vi "Process EMS Message.vi"(8 "error in (no error)":errorcluster, 10 "EMS Message":T1, 11 "Master Controller in":refnum<class "Master Controller.lvclass">) -> (0 "error out":errorcluster, 3 "Master Controller out":refnum<class "Master Controller.lvclass">)   [LabVIEW 2015, in "Master Controller Core.lvlib" / "Master Controller.lvclass"]
uses:
  Master Controller.lvclass
  Communications/SCADA Communcations Actor/SCADA Communications/Controls/EMS Message Cluster.ctl
  Master Controller.lvclass/Master Controller.ctl
  Communications/SCADA Communcations Actor/SCADA Communications Messages/Transmit EMS Message Msg/Transmit EMS Message Msg.lvclass/Transmit EMS Message Msg.ctl
  <vilib>/ActorFramework/Message Enqueuer/Message Enqueuer.lvclass/Message Enqueuer.ctl
  SCADA Core/SCADA Action Messages/Black Start Msg/Black Start Msg.lvclass/Black Start Msg.ctl
  <vilib>/ActorFramework/Actor/Actor.lvclass/Actor.ctl
  Master Controller Messages/Save CID File Msg/Save CID File Msg.lvclass/Save CID File Msg.ctl
  SCADA Core/SCADA Action Messages/Device Load Msg/Device Load Msg.lvclass/Device Load Msg.ctl
  SCADA Core/SCADA Action Messages/Device Unload Msg/Device Unload Msg.lvclass/Device Unload Msg.ctl
  IED Actor/IED/Controls/Device Activate Mode Select.ctl
  SCADA Core/SCADA Action Messages/Device Activate Msg/Device Activate Msg.lvclass/Device Activate Msg.ctl
  SCADA Core/SCADA Action Messages/Device Deactivate Msg/Device Deactivate Msg.lvclass/Device Deactivate Msg.ctl
  SCADA Core/SCADA Action Messages/Get Device Parameter Msg/Get Device Parameter Msg.lvclass/Get Device Parameter Msg.ctl
  SCADA Core/SCADA Action Messages/Set Device Parameter Msg/Set Device Parameter Msg.lvclass/Set Device Parameter Msg.ctl
  SCADA Core/SCADA Action Messages/Island Control Msg/Island Control Msg.lvclass/Island Control Msg.ctl
  SCADA Core/SCADA Action Messages/Get Measurement Msg/Get Measurement Msg.lvclass/Get Measurement Msg.ctl
  SCADA Core/SCADA Action Messages/Get Measurement (Multiple) Msg/Get Measurement (Multiple) Msg.lvclass/Get Measurement (Multiple) Msg.ctl
  SCADA Core/SCADA Action Messages/PCC Relay Msg/PCC Relay Msg.lvclass/PCC Relay Msg.ctl
  SCADA Core/SCADA Action Messages/Write Setpoint (Multiple) Msg/Write Setpoint (Multiple) Msg.lvclass/Write Setpoint (Multiple) Msg.ctl
  SCADA Core/SCADA Action Messages/Write Setpoint Msg/Write Setpoint Msg.lvclass/Write Setpoint Msg.ctl
  <vilib>/ActorFramework/Message Enqueuer/Enqueue.vi
  <vilib>/ActorFramework/Message Enqueuer/Init from Existing Queue.vi
  <vilib>/ActorFramework/Message Priority Queue/Priority Enqueue.vi
  Communications/SCADA Communcations Actor/SCADA Communications Messages/Transmit EMS Message Msg/Transmit EMS Message Msg.lvclass
  SCADA Core/SCADA Action Messages/Activate Msg/Activate Msg.lvclass
  SCADA Core/SCADA Action Messages/Black Start Msg/Black Start Msg.lvclass
  <vilib>/ActorFramework/Message Enqueuer/Message Enqueuer.lvclass
  Master Controller Messages/Save CID File Msg/Save CID File Msg.lvclass
  SCADA Core/SCADA Action Messages/Device Load Msg/Device Load Msg.lvclass
  SCADA Core/SCADA Action Messages/Device Unload Msg/Device Unload Msg.lvclass
  SCADA Core/SCADA Action Messages/Device Activate Msg/Device Activate Msg.lvclass
  SCADA Core/SCADA Action Messages/Device Deactivate Msg/Device Deactivate Msg.lvclass
  SCADA Core/SCADA Action Messages/Get Device Parameter Msg/Get Device Parameter Msg.lvclass
  SCADA Core/SCADA Action Messages/Set Device Parameter Msg/Set Device Parameter Msg.lvclass
  SCADA Core/SCADA Action Messages/Island Control Msg/Island Control Msg.lvclass
  SCADA Core/SCADA Action Messages/Get Measurement Msg/Get Measurement Msg.lvclass
  SCADA Core/SCADA Action Messages/Get Measurement (Multiple) Msg/Get Measurement (Multiple) Msg.lvclass
  SCADA Core/SCADA Action Messages/PCC Relay Msg/PCC Relay Msg.lvclass
  SCADA Core/SCADA Action Messages/Write Setpoint (Multiple) Msg/Write Setpoint (Multiple) Msg.lvclass
  SCADA Core/SCADA Action Messages/Write Setpoint Msg/Write Setpoint Msg.lvclass
  SCADA Core/SCADA Action Messages/Shutdown Msg/Shutdown Msg.lvclass
  SCADA Core/SCADA Action Messages/Synchronize Msg/Synchronize Msg.lvclass
  SCADA Core/SCADA Messages/Island Msg/Island Msg.lvclass
  Communications/SCADA Communcations Actor/SCADA Communications/SCADA Communications.lvclass
  <vilib>/ActorFramework/Actor/Actor.lvclass
  Utilities/Message Strings.llb/Message String Utilities.lvlib
  IED Actor/IED/IED.lvclass
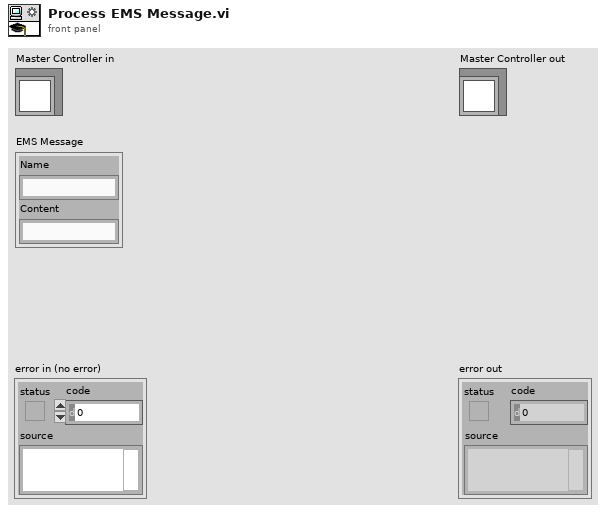
[diagram p1: front panel]
types:
  T1 = typedef "SCADA Communcations Actor.lvlib/SCADA Communications.lvclass/EMS Message Cluster.ctl" = cluster{"Name":string, "Content":string}
  T2 = typedef "IED Actor.lvlib/IED.lvclass/Device Activate Mode Select.ctl" = enum16{"Activate", "Blackstart", "Individual"}
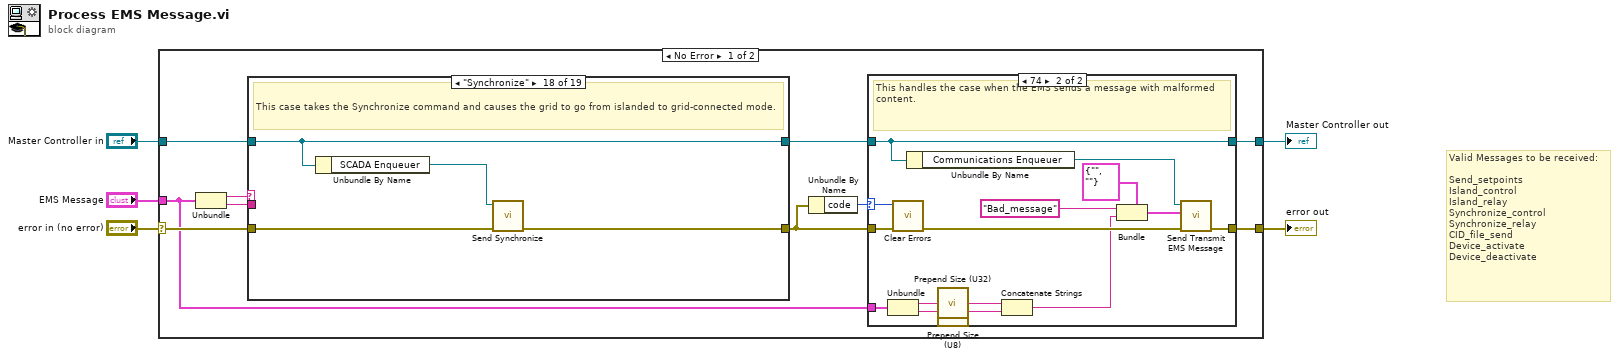
[diagram p0: block diagram]
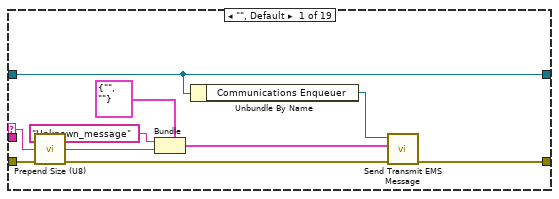
[diagram p3: hidden frame]
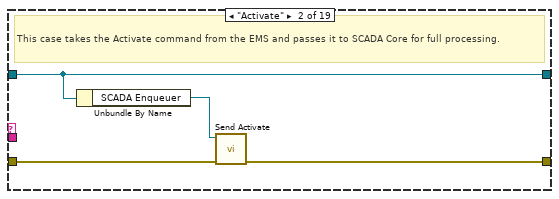
[diagram p4: hidden frame]
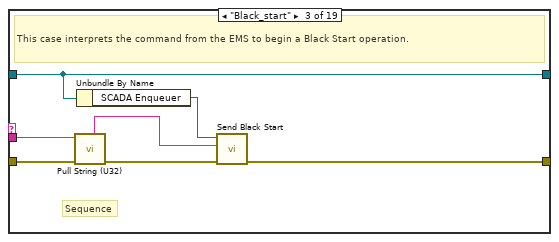
[diagram p5: hidden frame]
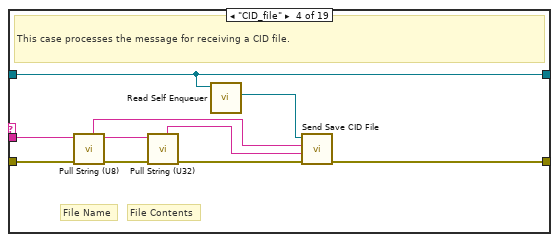
[diagram p6: hidden frame]
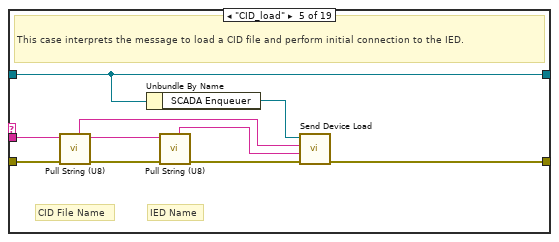
[diagram p7: hidden frame]
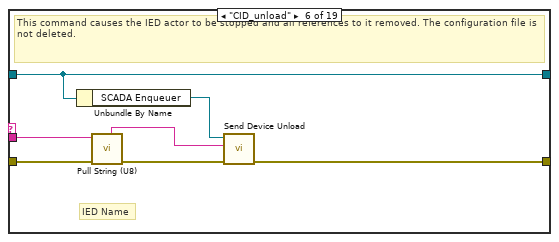
[diagram p8: hidden frame]
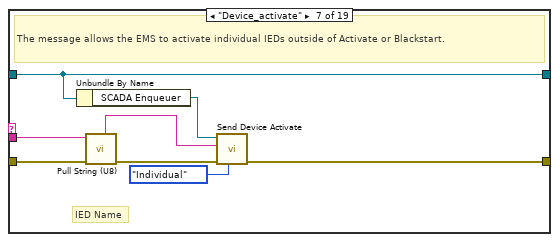
[diagram p9: hidden frame]
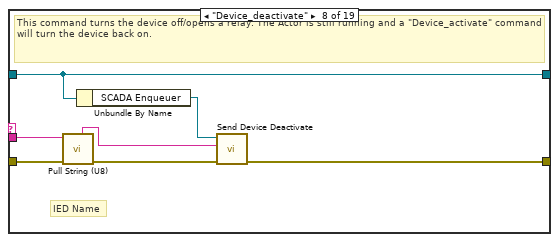
[diagram p10: hidden frame]
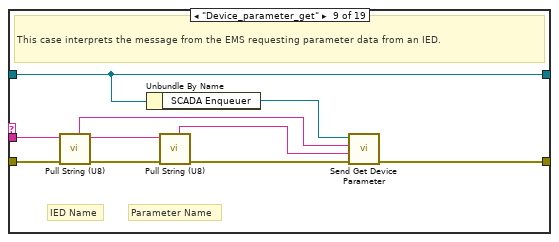
[diagram p11: hidden frame]
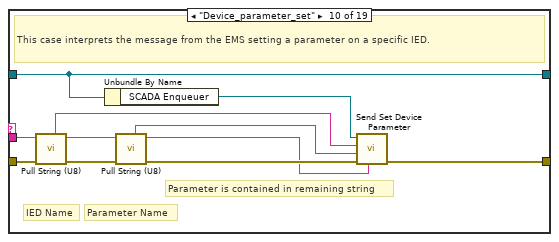
[diagram p12: hidden frame]
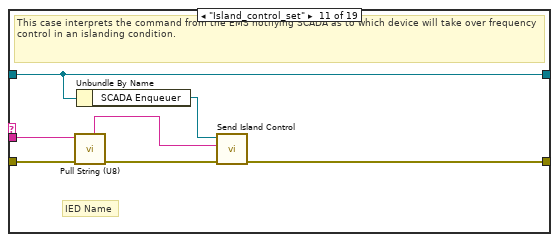
[diagram p13: hidden frame]
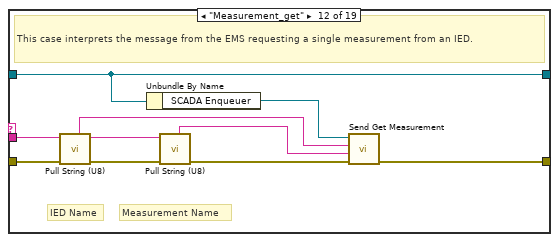
[diagram p14: hidden frame]
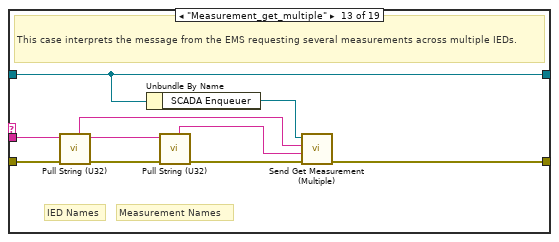
[diagram p15: hidden frame]
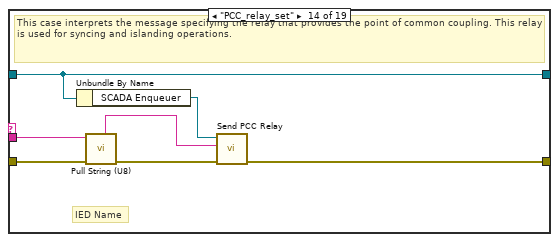
[diagram p16: hidden frame]
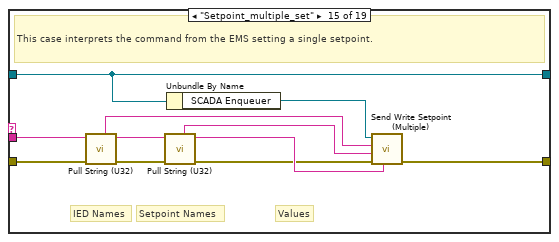
[diagram p17: hidden frame]
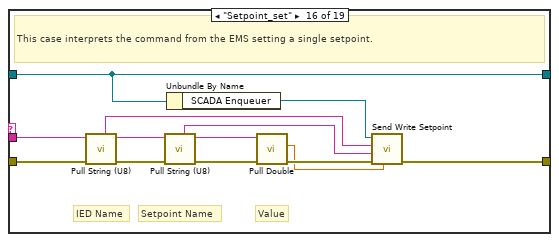
[diagram p18: hidden frame]
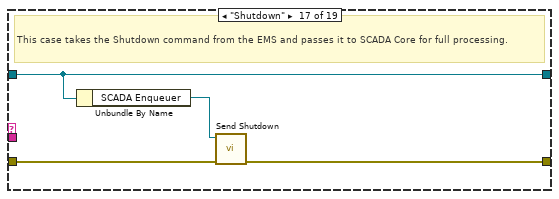
[diagram p19: hidden frame]
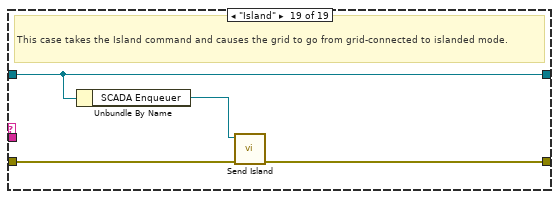
[diagram p20: hidden frame]
diagram:
  # "Valid Messages to be received:\n\nSend_setpoints\nIsland_control\nIsland_relay\nSynchronize_control\nSynchronize_relay\nCID_file_send\nDevice_activate\nDevice_deactivate"
  n1 = case shown="No Error" "error in (no error)" {
    selector: "error in (no error)" -> [w12 w187]
    tunnel: [w10 w187] -> w4
    tunnel: [w6 w186] -> w2
    tunnel: "Master Controller in" -> [w15 w186]
    tunnel: "EMS Message" -> [w8 _]
    frame No Error {
      n2 = Unbundle(w8) -> ("Name"=w14:string, "Content"=w13:string)
      n3 = case shown="\"Synchronize\"" w14 {
        selector: w14 -> [w35 _ _ _ _ _ _ _ _ _ _ _ _ _ _ _ _ _ _]
        tunnel: w15 -> [w41 w45 w52 w62 w72 w79 w87 w94 w104 w115 w122 w132 w142 w149 w160 w173 w177 w181 w185]
        tunnel: w13 -> [_ _ w49 w59 w68 w76 w84 w90 w102 w113 w119 w130 w140 w146 w157 w170 _ _ _]
        tunnel: [w41 w45 w52 w62 w72 w79 w87 w94 w104 w115 w122 w132 w142 w149 w160 w173 w177 w181 w185] -> w7
        tunnel: w12 -> [w36 w42 w48 w58 w69 w75 w83 w91 w103 w114 w118 w131 w141 w145 w156 w169 w174 w179 w183]
        tunnel: [w37 w43 w50 w60 w70 w78 w85 w92 w97 w108 w120 w125 w136 w147 w158 w171 w175 w178 w182] -> w9
        frame "", Default {
          n4 = call "Prepend Size (U8).vi"("String in"=w35) -> ("String out"=w33:string)
          n5 = Bundle(cluster=T1 {"Name"="", "Content"=""} ("Message"), "Name"="Unknown_message", "Content"=w33) -> (w38:T1)
          n6 = Unbundle By Name(w41) -> ("Communications Enqueuer"=w40:refnum<class "Message Enqueuer.lvclass">)
          n7 = call "Send Transmit EMS Message.vi"("error in (no error)"=w36, "Message"=w38, "Message Enqueuer"=w40) -> ("error out"=w37:errorcluster)  [unwired: 7 in, 1 out]
        }
        frame "Activate" {
          # "This case takes the Activate command from the EMS and passes it to SCADA Core for full processing."
          n8 = Unbundle By Name(w45) -> ("SCADA Enqueuer"=w44:refnum<class "Message Enqueuer.lvclass">)
          n9 = call "Send Activate.vi"("error in (no error)"=w42, "Message Enqueuer"=w44) -> ("error out"=w43:errorcluster)  [unwired: 8 in, 1 out]
        }
        frame "Black_start" {
          # "Sequence"
          # "This case interprets the command from the EMS to begin a Black Start operation."
          n10 = call "Pull String (U32).vi"("error in (no error)"=w48, "String in"=w49) -> ("error out"=w47:errorcluster, "String out"=w46:string)  [unwired: 7 in, 1 out]
          n11 = Unbundle By Name(w52) -> ("SCADA Enqueuer"=w51:refnum<class "Message Enqueuer.lvclass">)
          n12 = call "Send Black Start.vi"("error in (no error)"=w47, "Sequence"=w46, "Message Enqueuer"=w51) -> ("error out"=w50:errorcluster)  [unwired: 7 in, 1 out]
        }
        frame "CID_file" {
          # "File Contents"
          # "File Name"
          # "This case processes the message for receiving a CID file."
          n13 = call "Pull String (U8).vi"("error in (no error)"=w58, "String in"=w59) -> ("error out"=w56:errorcluster, "Remaining String"=w57:string, "String out"=w53:string)  [unwired: 7 in]
          n14 = call "Pull String (U32).vi"("error in (no error)"=w56, "String in"=w57) -> ("error out"=w55:errorcluster, "String out"=w54:string)  [unwired: 7 in, 1 out]
          n15 = call <vilib>:"Read Self Enqueuer.vi"("Actor"=w62) -> ("Self Enqueuer"=w61:refnum<class "Message Enqueuer.lvclass">)  [unwired: 10 in]
          n16 = call "Send Save CID File.vi"("error in (no error)"=w55, "Content"=w54, "File Name"=w53, "Message Enqueuer"=w61) -> ("error out"=w60:errorcluster)  [unwired: 6 in, 1 out]
        }
        frame "CID_load" {
          # "IED Name"
          # "CID File Name"
          # "This case interprets the message to load a CID file and perform initial connection to the IED."
          n17 = call "Pull String (U8).vi"("error in (no error)"=w69, "String in"=w68) -> ("error out"=w67:errorcluster, "Remaining String"=w63:string, "String out"=w65:string)  [unwired: 7 in]
          n18 = Unbundle By Name(w72) -> ("SCADA Enqueuer"=w71:refnum<class "Message Enqueuer.lvclass">)
          n19 = call "Pull String (U8).vi"("error in (no error)"=w67, "String in"=w63) -> ("error out"=w66:errorcluster, "String out"=w64:string)  [unwired: 7 in, 1 out]
          n20 = call "Send Device Load.vi"("error in (no error)"=w66, "IED Name"=w64, "CID File Name"=w65, "Message Enqueuer"=w71) -> ("error out"=w70:errorcluster)  [unwired: 6 in, 1 out]
        }
        frame "CID_unload" {
          # "IED Name"
          # "This command causes the IED actor to be stopped and all references to it removed. The configuration file is not deleted."
          n21 = Unbundle By Name(w79) -> ("SCADA Enqueuer"=w77:refnum<class "Message Enqueuer.lvclass">)
          n22 = call "Pull String (U8).vi"("error in (no error)"=w75, "String in"=w76) -> ("error out"=w74:errorcluster, "String out"=w73:string)  [unwired: 7 in, 1 out]
          n23 = call "Send Device Unload.vi"("error in (no error)"=w74, "IED Name"=w73, "Message Enqueuer"=w77) -> ("error out"=w78:errorcluster)  [unwired: 7 in, 1 out]
        }
        frame "Device_activate" {
          # "IED Name"
          # "The message allows the EMS to activate individual IEDs outside of Activate or Blackstart."
          n24 = Unbundle By Name(w87) -> ("SCADA Enqueuer"=w86:refnum<class "Message Enqueuer.lvclass">)
          n25 = call "Pull String (U8).vi"("error in (no error)"=w83, "String in"=w84) -> ("error out"=w82:errorcluster, "String out"=w81:string)  [unwired: 7 in, 1 out]
          n26 = call "Send Device Activate.vi"("Activate Mode"=Device_Activate_Mode_Select."Individual", "error in (no error)"=w82, "IED Name"=w81, "Message Enqueuer"=w86) -> ("error out"=w85:errorcluster)  [unwired: 6 in, 1 out]
        }
        frame "Device_deactivate" {
          # "IED Name"
          # "This command turns the device off/opens a relay. The Actor is still running and a \"Device_activate\" command will turn the device back on."
          n27 = call "Pull String (U8).vi"("error in (no error)"=w91, "String in"=w90) -> ("error out"=w89:errorcluster, "String out"=w88:string)  [unwired: 7 in, 1 out]
          n28 = Unbundle By Name(w94) -> ("SCADA Enqueuer"=w93:refnum<class "Message Enqueuer.lvclass">)
          n29 = call "Send Device Deactivate.vi"("error in (no error)"=w89, "IED Name"=w88, "Message Enqueuer"=w93) -> ("error out"=w92:errorcluster)  [unwired: 7 in, 1 out]
        }
        frame "Device_parameter_get" {
          # "Parameter Name"
          # "IED Name"
          # "This case interprets the message from the EMS requesting parameter data from an IED."
          n30 = call "Pull String (U8).vi"("error in (no error)"=w103, "String in"=w102) -> ("error out"=w101:errorcluster, "Remaining String"=w100:string, "String out"=w95:string)  [unwired: 7 in]
          n31 = Unbundle By Name(w104) -> ("SCADA Enqueuer"=w99:refnum<class "Message Enqueuer.lvclass">)
          n32 = call "Pull String (U8).vi"("error in (no error)"=w101, "String in"=w100) -> ("error out"=w98:errorcluster, "String out"=w96:string)  [unwired: 7 in, 1 out]
          n33 = call "Send Get Device Parameter.vi"("error in (no error)"=w98, "Parameter Name"=w96, "IED Name"=w95, "Message Enqueuer"=w99) -> ("error out"=w97:errorcluster)  [unwired: 6 in, 1 out]
        }
        frame "Device_parameter_set" {
          # "Parameter is contained in remaining string"
          # "Parameter Name"
          # "IED Name"
          # "This case interprets the message from the EMS setting a parameter on a specific IED."
          n34 = call "Pull String (U8).vi"("error in (no error)"=w114, "String in"=w113) -> ("error out"=w112:errorcluster, "Remaining String"=w111:string, "String out"=w106:string)  [unwired: 7 in]
          n35 = Unbundle By Name(w115) -> ("SCADA Enqueuer"=w110:refnum<class "Message Enqueuer.lvclass">)
          n36 = call "Pull String (U8).vi"("error in (no error)"=w112, "String in"=w111) -> ("error out"=w109:errorcluster, "Remaining String"=w105:string, "String out"=w107:string)  [unwired: 7 in]
          n37 = call "Send Set Device Parameter.vi"("Parameter"=w105, "error in (no error)"=w109, "Parameter Name"=w107, "IED Name"=w106, "Message Enqueuer"=w110) -> ("error out"=w108:errorcluster)  [unwired: 5 in, 1 out]
        }
        frame "Island_control_set" {
          # "IED Name"
          # "This case interprets the command from the EMS notifying SCADA as to which device will take over frequency control in an islanding condition."
          n38 = call "Pull String (U8).vi"("error in (no error)"=w118, "String in"=w119) -> ("error out"=w117:errorcluster, "String out"=w116:string)  [unwired: 7 in, 1 out]
          n39 = Unbundle By Name(w122) -> ("SCADA Enqueuer"=w121:refnum<class "Message Enqueuer.lvclass">)
          n40 = call "Send Island Control.vi"("error in (no error)"=w117, "IED Name"=w116, "Message Enqueuer"=w121) -> ("error out"=w120:errorcluster)  [unwired: 7 in, 1 out]
        }
        frame "Measurement_get" {
          # "Measurement Name"
          # "IED Name"
          # "This case interprets the message from the EMS requesting a single measurement from an IED."
          n41 = call "Pull String (U8).vi"("error in (no error)"=w131, "String in"=w130) -> ("error out"=w129:errorcluster, "Remaining String"=w128:string, "String out"=w123:string)  [unwired: 7 in]
          n42 = Unbundle By Name(w132) -> ("SCADA Enqueuer"=w127:refnum<class "Message Enqueuer.lvclass">)
          n43 = call "Pull String (U8).vi"("error in (no error)"=w129, "String in"=w128) -> ("error out"=w126:errorcluster, "String out"=w124:string)  [unwired: 7 in, 1 out]
          n44 = call "Send Get Measurement.vi"("error in (no error)"=w126, "Measurement Name"=w124, "IED Name"=w123, "Message Enqueuer"=w127) -> ("error out"=w125:errorcluster)  [unwired: 6 in, 1 out]
        }
        frame "Measurement_get_multiple" {
          # "Measurement Names"
          # "IED Names"
          # "This case interprets the message from the EMS requesting several measurements across multiple IEDs."
          n45 = call "Pull String (U32).vi"("error in (no error)"=w141, "String in"=w140) -> ("error out"=w139:errorcluster, "Remaining String"=w138:string, "String out"=w134:string)  [unwired: 7 in]
          n46 = Unbundle By Name(w142) -> ("SCADA Enqueuer"=w135:refnum<class "Message Enqueuer.lvclass">)
          n47 = call "Pull String (U32).vi"("error in (no error)"=w139, "String in"=w138) -> ("error out"=w137:errorcluster, "String out"=w133:string)  [unwired: 7 in, 1 out]
          n48 = call "Send Get Measurement (Multiple).vi"("error in (no error)"=w137, "Measurement Names"=w133, "IED Names"=w134, "Message Enqueuer"=w135) -> ("error out"=w136:errorcluster)  [unwired: 6 in, 1 out]
        }
        frame "PCC_relay_set" {
          # "IED Name"
          # "This case interprets the message specifying the relay that provides the point of common coupling. This relay is used for syncing and islanding operations."
          n49 = Unbundle By Name(w149) -> ("SCADA Enqueuer"=w148:refnum<class "Message Enqueuer.lvclass">)
          n50 = call "Pull String (U8).vi"("error in (no error)"=w145, "String in"=w146) -> ("error out"=w144:errorcluster, "String out"=w143:string)  [unwired: 7 in, 1 out]
          n51 = call "Send PCC Relay.vi"("error in (no error)"=w144, "Relay Name"=w143, "Message Enqueuer"=w148) -> ("error out"=w147:errorcluster)  [unwired: 7 in, 1 out]
        }
        frame "Setpoint_multiple_set" {
          # "Values"
          # "Setpoint Names"
          # "IED Names"
          # "This case interprets the command from the EMS setting a single setpoint."
          n52 = call "Pull String (U32).vi"("error in (no error)"=w156, "String in"=w157) -> ("error out"=w155:errorcluster, "Remaining String"=w154:string, "String out"=w152:string)  [unwired: 7 in]
          n53 = call "Pull String (U32).vi"("error in (no error)"=w155, "String in"=w154) -> ("error out"=w150:errorcluster, "Remaining String"=w151:string, "String out"=w153:string)  [unwired: 7 in]
          n54 = Unbundle By Name(w160) -> ("SCADA Enqueuer"=w159:refnum<class "Message Enqueuer.lvclass">)
          n55 = call "Send Write Setpoint (Multiple).vi"("Values"=w151, "error in (no error)"=w150, "Variables"=w153, "IED Names"=w152, "Message Enqueuer"=w159) -> ("error out"=w158:errorcluster)  [unwired: 5 in, 1 out]
        }
        frame "Setpoint_set" {
          # "Value"
          # "Setpoint Name"
          # "IED Name"
          # "This case interprets the command from the EMS setting a single setpoint."
          n56 = call "Pull String (U8).vi"("error in (no error)"=w169, "String in"=w170) -> ("error out"=w168:errorcluster, "Remaining String"=w167:string, "String out"=w162:string)  [unwired: 7 in]
          n57 = call "Pull String (U8).vi"("error in (no error)"=w168, "String in"=w167) -> ("error out"=w166:errorcluster, "Remaining String"=w165:string, "String out"=w163:string)  [unwired: 7 in]
          n58 = Unbundle By Name(w173) -> ("SCADA Enqueuer"=w172:refnum<class "Message Enqueuer.lvclass">)
          n59 = call "Pull Double.vi"("error in (no error)"=w166, "String in"=w165) -> ("error out"=w164:errorcluster, "Double out"=w161:dbl)  [unwired: 7 in, 1 out]
          n60 = call "Send Write Setpoint.vi"("Value"=w161, "error in (no error)"=w164, "Variable"=w163, "IED Name"=w162, "Message Enqueuer"=w172) -> ("error out"=w171:errorcluster)  [unwired: 5 in, 1 out]
        }
        frame "Shutdown" {
          # "This case takes the Shutdown command from the EMS and passes it to SCADA Core for full processing."
          n61 = Unbundle By Name(w177) -> ("SCADA Enqueuer"=w176:refnum<class "Message Enqueuer.lvclass">)
          n62 = call "Send Shutdown.vi"("error in (no error)"=w174, "Message Enqueuer"=w176) -> ("error out"=w175:errorcluster)  [unwired: 8 in, 1 out]
        }
        frame "Synchronize" {
          # "This case takes the Synchronize command and causes the grid to go from islanded to grid-connected mode."
          n63 = Unbundle By Name(w181) -> ("SCADA Enqueuer"=w180:refnum<class "Message Enqueuer.lvclass">)
          n64 = call "Send Synchronize.vi"("error in (no error)"=w179, "Message Enqueuer"=w180) -> ("error out"=w178:errorcluster)  [unwired: 8 in, 1 out]
        }
        frame "Island" {
          # "This case takes the Island command and causes the grid to go from grid-connected to islanded mode."
          n65 = Unbundle By Name(w185) -> ("SCADA Enqueuer"=w184:refnum<class "Message Enqueuer.lvclass">)
          n66 = call "Send Island.vi"("error in (no error)"=w183, "Message Enqueuer"=w184) -> ("error out"=w182:errorcluster)  [unwired: 8 in, 1 out]
        }
      }
      n67 = Unbundle By Name(w9) -> ("code"=w11:i32)
      n68 = case shown="74" w11 {
        selector: w11 -> [_ w26]
        tunnel: [w17 w30] -> w10
        tunnel: w9 -> [w17 w25]
        tunnel: w8 -> [_ w23]
        tunnel: w7 -> [w16 w32]
        tunnel: [w16 w32] -> w6
        frame 0, Default {
        }
        frame 74 {
          # "This handles the case when the EMS sends a message with malformed content."
          n69 = Unbundle(w23) -> ("Name"=w22:string, "Content"=w21:string)
          n70 = call <vilib>:"Clear Errors.vi"("error in (no error)"=w25, "specific error code to clear (0: all)"=w26) -> ("error out"=w24:errorcluster)  [unwired: 4 in, 1 out]
          n71 = Unbundle By Name(w32) -> ("Communications Enqueuer"=w31:refnum<class "Message Enqueuer.lvclass">)
          n72 = call "Prepend Size (U8).vi"("String in"=w22) -> ("String out"=w20:string)
          n73 = call "Prepend Size (U32).vi"("String in"=w21) -> ("String out"=w19:string)
          n74 = Concatenate Strings(w20, w19) -> (w18:string)
          n75 = Bundle(cluster=T1 {"Name"="", "Content"=""} ("Message"), "Name"="Bad_message", "Content"=w18) -> (w28:T1)
          n76 = call "Send Transmit EMS Message.vi"("error in (no error)"=w24, "Message"=w28, "Message Enqueuer"=w31) -> ("error out"=w30:errorcluster)  [unwired: 7 in, 1 out]
        }
      }
    }
    frame Error {
    }
  }
  "error out" <- w4
  "Master Controller out" <- w2
